vi "Configure Channels.vi"(8 "error in":errorcluster, 11 "Thermometer DAQmx RTD Cont CFG in":refnum<class "Thermometer DAQmx TC Cont CFG.lvclass">) -> (0 "error out":errorcluster, 3 "Thermometer DAQmx RTD Cont CFG out":refnum<class "Thermometer DAQmx TC Cont CFG.lvclass">)   [LabVIEW 2024, in "Thermometer DAQmx TC Cont CFG.lvclass"]
uses:
  Thermometer DAQmx TC Cont CFG.lvclass
  D:/git/HAL/HAL/Configurations/CFG JSON/CFG JSON.lvclass
  D:/git/HAL/HAL/Devices/DAQmx/DAQmx Base CFG/DAQmx Base CFG.lvclass
  D:/git/HAL/HAL/Configurations/CFG Base/CFG Base.lvclass
  Thermometer DAQmx TC Cont CFG.lvclass/Thermometer DAQmx TC Cont CFG.ctl
  DAQmx Base CFG/DAQmx Base CFG.lvclass/DAQmx Base CFG.ctl
  Configurations/CFG Base/CFG Base.lvclass/CFG Base.ctl
  3c552e12-cc6d-4feb-bdfa-5cb71c1a3aaa.vi
  3c552e12-cc6d-4feb-bdfa-5cb71c1a3aaa.vi/a4169a97-72fc-4003-a778-603cf20cafa0.vi
  <vilib>/JDP Science/JSONtext/Find Item.vi
  <vilib>/JDP Science/JSONtext/Next JSON Value.vi
  <vilib>/JDP Science/JSONtext/String Subset.vi
  <vilib>/JDP Science/JSONtext/Parsing/Advance past next JSON Value (inlined COPY).vi
  <vilib>/JDP Science/JSONtext/Parsing/Advance past whitespace.vi
  <vilib>/JDP Science/JSONtext/Parsing/Advance past String.vi
  <vilib>/JDP Science/JSONtext/Parsing/Advance past Number.vi
  <vilib>/JDP Science/JSONtext/Parsing/Advance past Line Ending.vi
  <vilib>/JDP Science/JSONtext/Parsing/Parse Full Path or Item Name.vi
  <vilib>/JDP Science/JSONtext/Parsing/Advance past Array.vi
  <vilib>/JDP Science/JSONtext/Parsing/Advance past Object.vi
  <vilib>/JDP Science/JSONtext/support/Error Cluster From Code.vi
  <vilib>/JDP Science/JSONtext/Offset/Find Item Locations by Path.vi
  <vilib>/JDP Science/JSONtext/JSON text to Variant.vi
  <vilib>/Utility/error.llb/Error Cluster From Error Code.vi
  <vilib>/DAQmx/create/channels.llb/DAQmx Create Channel (AI-Temperature-Thermocouple).vi
  <vilib>/JDP Science/JSONtext/LVClass Serializer/JSONtext LVClass Serializer.lvclass
  DAQmx Base CFG/DAQmx Base CFG.lvclass
  Configurations/CFG JSON/CFG JSON.lvclass
  Buffers/BufferLastReadingsDBL/BufferLastReadsDBL.lvclass
  Configurations/CFG Base/CFG Base.lvclass
panel:
  out "thermocouple type":i32(ring)=10072 items=["J"=10072, "K"=10073, "N"=10077, "R"=10082, "S"=10085, "T"=10086, "B"=10047, "E"=10055]
  out "cjc source":i32(ring)=10116 items=["Built-In"=10200, "Constant Value"=10116, "Channel"=10113]
  out "units":i32(ring)=10143 items=["Deg C"=10143, "Deg F"=10144, "Kelvins"=10325, "Deg R"=10145, "From Custom Scale"=10065]
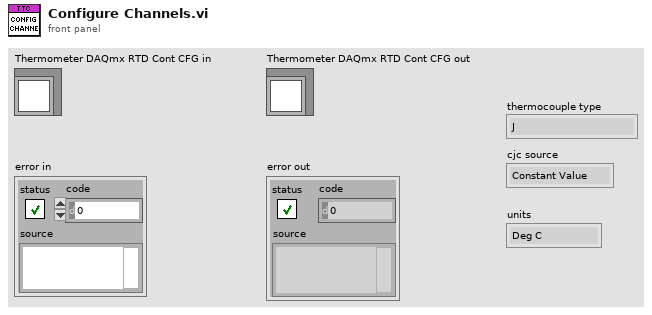
[diagram p1: front panel]
types:
  T1 = cluster{"Name":string, "Enabled":bool, "Minimum Value":dbl, "Maximum Value":dbl, "Thermocouple Type":string, "Units":string, "CJC Channel":string, "CJC Source":string, "CJC Value":dbl}[]
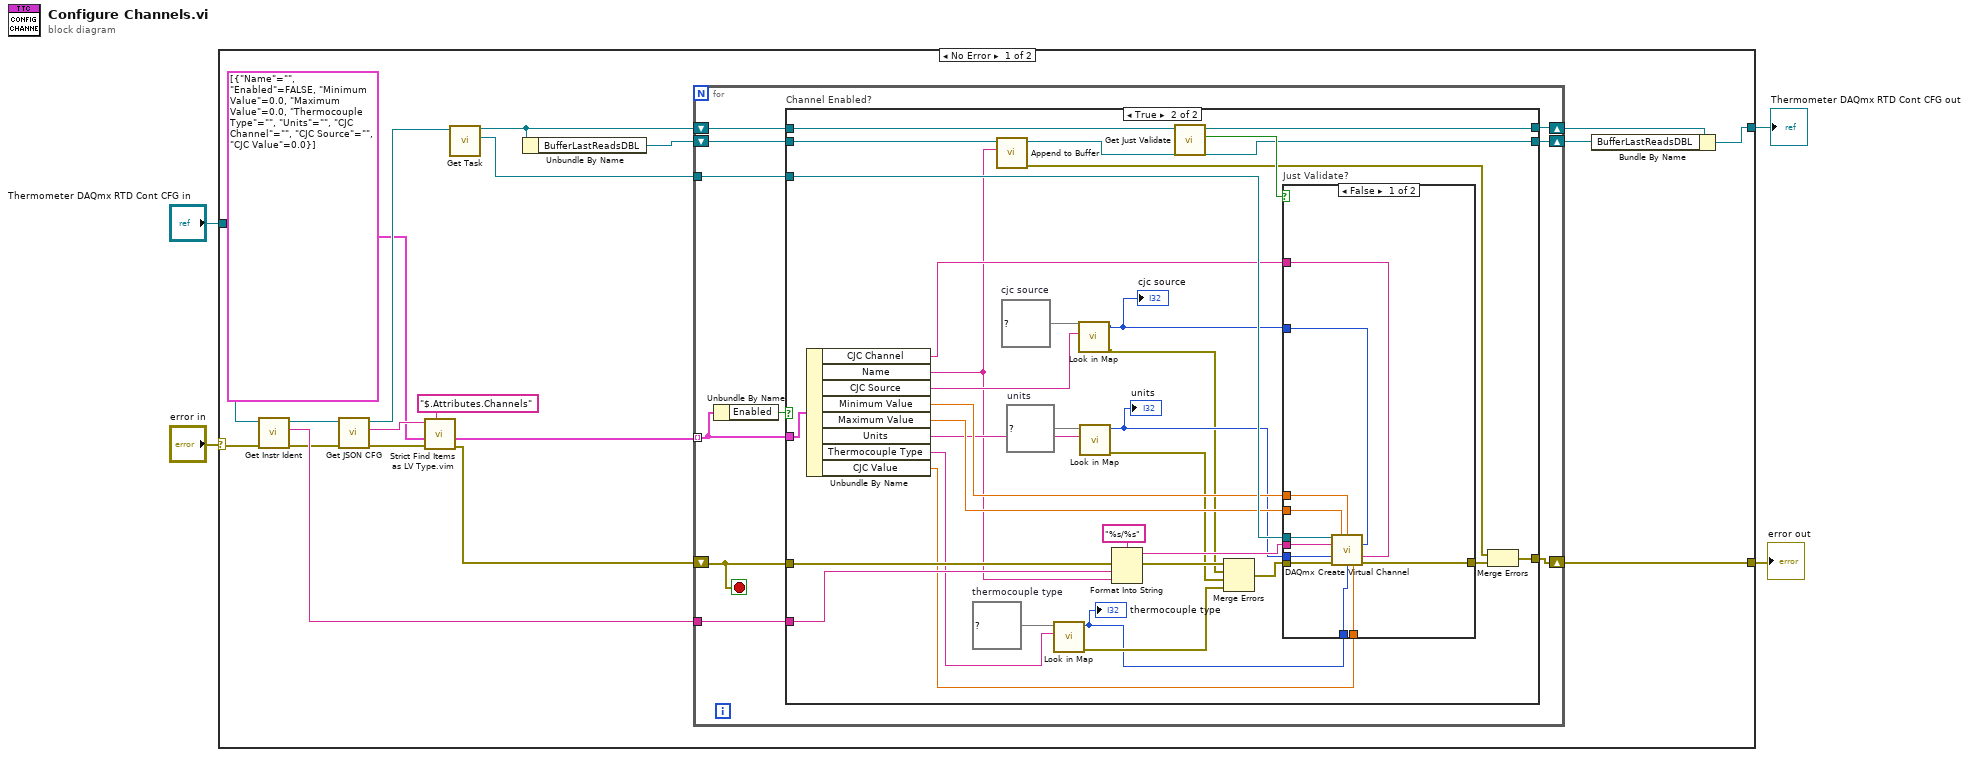
[diagram p0: block diagram]
diagram:
  n1 = case shown="No Error" "error in" {
    selector: "error in" -> [w19 w81]
    tunnel: "Thermometer DAQmx RTD Cont CFG in" -> [w17 w82]
    tunnel: [w20 w81] -> w1
    tunnel: [w6 w82] -> w2
    frame No Error {
      n2 = call-dynamic "Get Instr Ident.vi"("error in"=w19, "CFG JSON in"=w17) -> ("error out"=w15:errorcluster, "Instr Ident"=w21:string, "CFG JSON out"=w22:refnum<class "Thermometer DAQmx TC Cont CFG.lvclass">)  [unwired: 7 in]
      n3 = call "Get JSON CFG.vi"("CFG JSON in"=w22) -> ("<JSON> CFG"=w14:string, "CFG JSON out"=w16:refnum<class "Thermometer DAQmx TC Cont CFG.lvclass">)  [unwired: 9 in]
      n4 = call "Strict Find Items as LV Type.vim"("$Path or Item Name"="$.Attributes.Channels", "error in"=w15, "Data Type and Default Value"=T1 [{"Name"="", "Enabled"=FALSE, "Minimum Value"=0.0, "Maximum Value"=0.0, "Thermocouple Type"="", "Units"="", "CJC Channel"="", "CJC Source"="", "CJC Value"=0.0}], "<JSON>"=w14) -> ("error out"=w11:errorcluster, "Data out"=w10:T1)  [unwired: 5 in, 1 out]
      n5 = call "Get Task.vi"("DAQmx Base CFG in"=w16) -> ("Task"=w18:refnum<k21>, "DAQmx Base CFG out"=w9:refnum<class "Thermometer DAQmx TC Cont CFG.lvclass">)  [unwired: 9 in]
      n6 = Unbundle By Name(w9) -> ("BufferLastReadsDBL"=w8:refnum<class "BufferLastReadsDBL.lvclass">)
      n7 = for {
        tunnel: w10 -> [w29] mode=indexing
        shift-right: [w32] -> w20
        shift-left: w11 -> [w31]
        tunnel: w21 -> [w30]
        tunnel: w18 -> [w28]
        shift-right: [w27] -> w7
        shift-left: w9 -> [w26]
        shift-right: [w23] -> w5
        shift-left: w8 -> [w24]
        stop <- w31 stop-if-true
        n8 = Unbundle By Name(w29) -> ("Enabled"=w25:bool)
        n9 = case "Channel Enabled?" shown="True" w25 {
          tunnel: [w35 w37] -> w32
          tunnel: w31 -> [w35 w65]
          tunnel: w30 -> [_ w64]
          tunnel: w29 -> [_ w68]
          tunnel: [w34 w40] -> w27
          tunnel: w28 -> [_ w67]
          tunnel: w26 -> [w34 w42]
          tunnel: w24 -> [w33 w43]
          tunnel: [w33 w39] -> w23
          frame False {
          }
          frame True {
            w49 = map{string, i32} {"B"=10047, "E"=10055, "J"=10072, "K"=10073, "N"=10077, "R"=10082, "S"=10085, "T"=10086}  # thermocouple type
            w50 = map{string, i32} {"Built-In"=10200, "Channel"=10113, "Constant Value"=10116}  # cjc source
            w58 = map{string, i32} {"Deg C"=10143, "Deg F"=10144, "Deg R"=10145, "From Custom Scale"=10065, "Kelvins"=10325}  # units
            n10 = Unbundle By Name(w68) -> ("CJC Channel"=w45:string, "Name"=w44:string, "CJC Source"=w52:string, "Minimum Value"=w60:dbl, "Maximum Value"=w59:dbl, "Units"=w56:string, "Thermocouple Type"=w54:string, "CJC Value"=w46:dbl)
            n11 = call "Append to Buffer.vi"("Channel"=w44, "BufferLastReadingsDBL in"=w43) -> ("error out"=w36:errorcluster, "BufferLastReadingsDBL out"=w39:refnum<class "BufferLastReadsDBL.lvclass">)  [unwired: 8 in]
            n12 = call "Look in Map.vi"("Key"=w54, "Map"=w49) -> ("error out"=w53:errorcluster, "Value"=w47:i32)  [unwired: 8 in]
            "thermocouple type" <- w47
            n13 = call "Look in Map.vi"("Key"=w52, "Map"=w50) -> ("error out"=w51:errorcluster, "Value"=w48:i32)  [unwired: 8 in]
            "cjc source" <- w48
            n14 = call "Look in Map.vi"("Key"=w56, "Map"=w58) -> ("error out"=w55:errorcluster, "Value"=w57:i32)  [unwired: 8 in]
            "units" <- w57
            n15 = Format Into String(format string="%s/%s", error in=w65, w64, w44) -> (resulting string=w62:string, error out=w63:errorcluster)  [unwired: 1 in]
            n16 = call "Get Just Validate.vi"("CFG Base in"=w42) -> ("Just Validate"=w41:bool, "CFG Base out"=w40:refnum<class "Thermometer DAQmx TC Cont CFG.lvclass">)  [unwired: 9 in]
            n17 = Merge Errors(w63, w51, w55, w53) -> (w61:errorcluster)
            n18 = case "Just Validate?" shown="False" w41 {
              tunnel: w61 -> [w72 w80]
              tunnel: w62 -> [w77 _]
              tunnel: w67 -> [w79 _]
              tunnel: [w78 w80] -> w38
              tunnel: w48 -> [w74 _]
              tunnel: w60 -> [w76 _]
              tunnel: w59 -> [w75 _]
              tunnel: w57 -> [w73 _]
              tunnel: w47 -> [w70 _]
              tunnel: w46 -> [w71 _]
              tunnel: w45 -> [w69 _]
              frame False {
                n19 = call-poly <vilib>:"DAQmx Create Virtual Channel.vi"("task in"=w79, "maximum value"=w75, "minimum value"=w76, "physical channels"=w77, "cjc source"=w74, "units"=w73, "cjc channel"=w69, "error in"=w72, "thermocouple type"=w70, "cjc value"=w71) -> ("error out"=w78:errorcluster)  [unwired: 4 in, 1 out]
              }
              frame True {
              }
            }
            n20 = Merge Errors(w36, w38) -> (w37:errorcluster)
          }
        }
      }
      n21 = Bundle By Name(cluster=w7, "BufferLastReadsDBL"=w5) -> (w6:refnum<class "Thermometer DAQmx TC Cont CFG.lvclass">)
    }
    frame Error {
    }
  }
  "error out" <- w1
  "Thermometer DAQmx RTD Cont CFG out" <- w2
